vi "TCPIP IO.vi"(4 "error in (no error)":errorcluster, 5 "TCP TMO\n(10000 ms)":i32=10000, 7 "Commands":cluster{"Command":string, "Params":variant[]}[](array[cluster])) -> (0 "error out":errorcluster, 3 "Responses":cluster{string, variant[]}[](array[cluster]))   [LabVIEW 2011]
uses:
  HWIO Global.vi
panel:
  out "LoopTime (ms)":u32
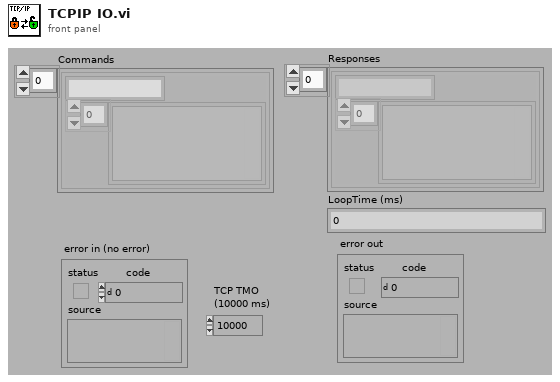
[diagram p1: front panel]
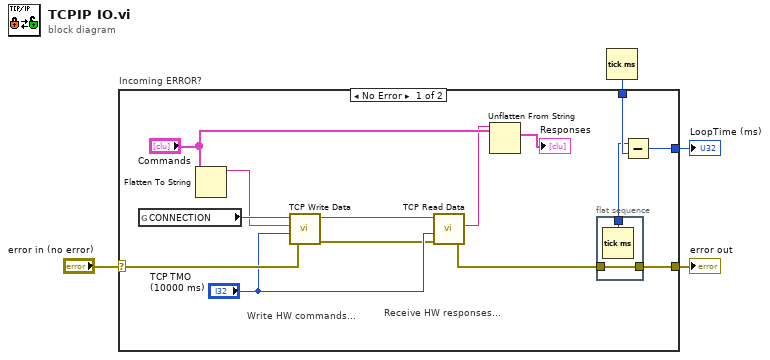
[diagram p0: block diagram]
diagram:
  n1 = Tick Count (ms)() -> (millisecond timer value=w3:u32)
  n2 = case "Incoming ERROR?" shown="No Error" "error in (no error)" {
    selector: "error in (no error)" -> [w18 w21]
    tunnel: [w5 w21] -> w1
    tunnel: w3 -> [w9 _]
    tunnel: [w7 _] -> w2
    frame No Error {
      # "Receive HW responses..."
      # "Write HW commands..."
      n3 = global read "HWIO Global.vi" "CONNECTION"() -> (w15:refnum<k5>)
      n4 = Flatten To String(anything="Commands") -> (data string=w14:string)  [unwired: 1 in, 4 out]
      n5 = call "TCP Write Data.vi"("error in (no error)"=w18, "timeout ms (25000)"="TCP TMO\n(10000 ms)", "Flattened Data"=w14, "connection ID"=w15) -> ("error out"=w10:errorcluster, "dup connection ID"=w12:refnum<k5>)  [unwired: 2 out]
      n6 = call "TCP Read Data.vi"("error in (no error)"=w10, "Timeout (25000 ms)"="TCP TMO\n(10000 ms)", "connection ID"=w12) -> ("error out"=w6:errorcluster, "Flat Data"=w13:string)  [unwired: 3 out]
      n7 = Unflatten From String(type="Commands", binary string=w13) -> (value=→"Responses":cluster{"Command":string, "Params":variant[]}[])  [unwired: 1 in, 4 out]
      n8 = flat-sequence {
        tunnel: [w20] -> w8
        tunnel: w6 -> [w19]
        tunnel: [w19] -> w5
        frame #0 {
          n9 = Tick Count (ms)() -> (millisecond timer value=w20:u32)
        }
      }
      n10 = Subtract(x=w8, y=w9) -> (x-y=w7:u32)
    }
    frame Error {
    }
  }
  "error out" <- w1
  "LoopTime (ms)" <- w2
